vi "Mysql data reader 2D double.vi"(8 "error in (no error)":errorcluster, 11 ".NET Refnum in":refnum<k24>) -> (0 "error out":errorcluster, 3 "Array":dbl[][](array[numeric]))   [LabVIEW 2020, in "mysql.lvlib" / "mysql.lvclass"]
uses:
  mysql.lvclass
  MySql.Data
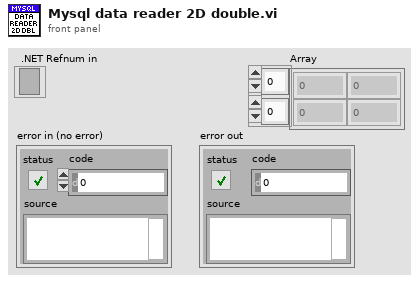
[diagram p1: front panel]
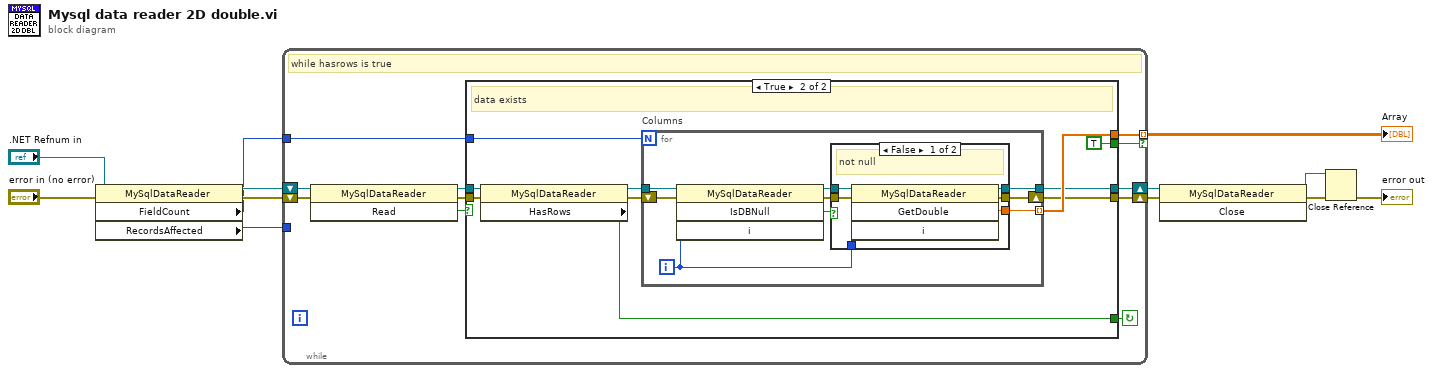
[diagram p0: block diagram]
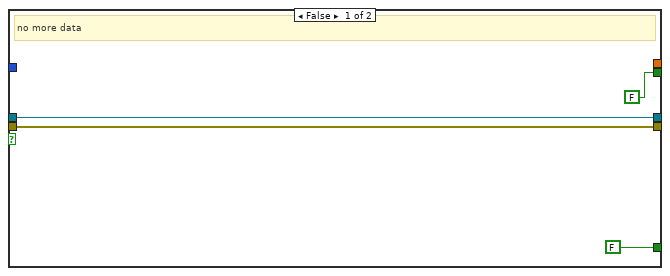
[diagram p2: hidden frame]
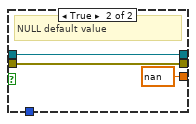
[diagram p3: hidden frame]
diagram:
  n1 = property class="MySqlDataReader"(reference=".NET Refnum in", error in="error in (no error)") -> (reference out=w7:refnum<k24>, error out=w6:errorcluster, "FieldCount"=w3:i32, "RecordsAffected"=w12:i32)
  n2 = while {
    tunnel: w3 -> [w23]
    tunnel: [w22] -> w4 mode=indexing if=w13
    shift-right: [w16] -> w9
    shift-left: w6 -> [w21]
    shift-right: [w17] -> w8
    shift-left: w7 -> [w19]
    tunnel: w12 -> [_]
    stop <- w15 continue-if-true
    # "while hasrows is true"
    n3 = invoke class="MySqlDataReader" method="Read"(reference=w19, error in=w21) -> (reference out=w18:refnum<k24>, error out=w20:errorcluster, "Read"=w14:bool)  [unwired: 1 in]
    n4 = case shown="True" w14 {
      tunnel: w23 -> [_ w37]
      tunnel: [_ w36] -> w22
      tunnel: w20 -> [w25 w35]
      tunnel: w18 -> [w26 w34]
      tunnel: [w26 w33] -> w17
      tunnel: [w25 w29] -> w16
      tunnel: [FALSE ("HasRows") w30] -> w15
      tunnel: [FALSE TRUE] -> w13
      frame False {
        # "no more data"
      }
      frame True {
        # "data exists"
        n5 = property class="MySqlDataReader"(reference=w34, error in=w35) -> (reference out=w32:refnum<k24>, error out=w31:errorcluster, "HasRows"=w30:bool)
        n6 = for "Columns" {
          N: w37 -> [_]
          tunnel: w32 -> [w41]
          shift-right: [w46] -> w29
          shift-left: w31 -> [w42]
          tunnel: [w45] -> w36 mode=indexing
          tunnel: [w44] -> w33
          i -> [w43]
          n7 = invoke class="MySqlDataReader" method="IsDBNull"(reference=w41, error in=w42, "i"=w43) -> (reference out=w40:refnum<k24>, error out=w39:errorcluster, "IsDBNull"=w38:bool)  [unwired: 1 in, 1 out]
          n8 = case shown="False" w38 {
            tunnel: [w52 w54] -> w46
            tunnel: [w51 nan ("GetDouble")] -> w45
            tunnel: [w50 w55] -> w44
            tunnel: w43 -> [w49 _]
            tunnel: w40 -> [w48 w55]
            tunnel: w39 -> [w47 w54]
            frame False {
              # "not null"
              n9 = invoke class="MySqlDataReader" method="GetDouble"(reference=w48, error in=w47, "i"=w49) -> (reference out=w50:refnum<k24>, error out=w52:errorcluster, "GetDouble"=w51:dbl)  [unwired: 1 in, 1 out]
            }
            frame True {
              # "NULL default value"
            }
          }
        }
      }
    }
  }
  "Array" <- w4
  n10 = invoke class="MySqlDataReader" method="Close"(reference=w8, error in=w9) -> (reference out=w11:refnum<k24>, error out=w10:errorcluster)  [unwired: 1 in, 1 out]
  n11 = Close Reference(reference=w11, error in (no error)=w10) -> (error out=→"error out":errorcluster)
